vi "Logging Active.vi"(8 "error in (no error)":errorcluster, 11 "Active in":refnum<class "Active.lvclass">) -> (0 "error out":errorcluster, 3 "_State Machine Actor out":refnum<class "_State Machine Actor.lvclass">)   [LabVIEW 2024, in "Active.lvlib" / "Active.lvclass"]
uses:
  Active.lvclass
  _State Machine Actor/_State Machine Actor/_State Machine Actor.lvclass
  Logging/Logging/Logging.lvclass
  C:/Users/uspoaotto/OneDrive - Oregon Tool/Desktop/working copies/stateMachineActor/src/_State Machine Actor/_State Machine Actor/_State Machine Actor.lvclass
  Active.lvclass/Active.ctl
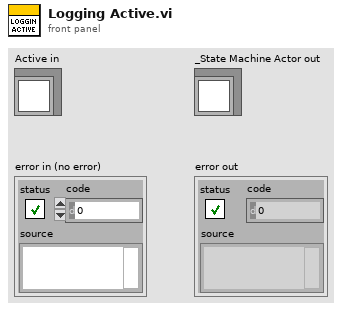
[diagram p1: front panel]
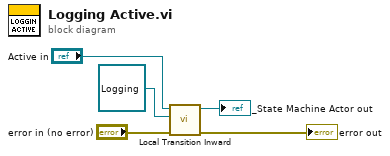
[diagram p0: block diagram]
diagram:
  n1 = call-dynamic "Local Transition Inward.vi"("error in (no error)"="error in (no error)", "Target State"=refnum<class "Logging.lvclass"> refnum ("Logging.lvlib:Logging.lvclass"), "State Machine Actor in"="Active in") -> ("error out"=→"error out":errorcluster, "_State Machine Actor out"=→"_State Machine Actor out":refnum<class "_State Machine Actor.lvclass">)  [unwired: 7 in]
